vi "Ecal.vi"(0 "VISA IN":refnum<visa-resource-name>="GPIB1::16::INSTR", 5 "error in":errorcluster) -> (14 "VISA Out":refnum<visa-resource-name>="GPIB1::16::INSTR", 19 "error out":errorcluster)   [LabVIEW 2018, in "PNA-X.lvlib"]
doc: "' Performing a 2-port cal (Ports 1 and 2)\nDim app\nDim scpi\n\n' Create / Get the PNA application.\nSet app = CreateObject(\"AgilentPNA835x.Application\")\nSet scpi = app.ScpiStringParser\n\n' Specify the DUT connectors\n' (for each connector of your DUT, one of the ECal module's ports must have\n' that same connector, or else you cannot achieve the cal using that module).\nscpi.Execute \"sens:corr:coll:guid:conn:port1 \"\"APC 3.5 female\"\" \"\nscpi.Execute \"sens:corr:coll:guid:conn:port2 \"\"APC 3.5 male\"\" \"\n\n' Note: If your PNA has more than 2 ports, you would need to uncomment\n' one or both of these next two lines, to explicitly specify this is\n' just a 2-port cal.\n'scpi.Execute \"sens:corr:coll:guid:conn:port3 \"\"Not used\"\" \"\n'scpi.Execute \"sens:corr:coll:guid:conn:port4 \"\"Not used\"\" \"\nMsgBox \"Connectors defined for Ports 1 and 2\" \n\n' Select the ECal module for each port being calibrated.\n' Replace N4691-60004 with the part number printed on your module\n' followed by User x if using a User characterization, then the word 'ECal'\n' Your ECal module must already be connected via USB to the PNA.\nscpi.Execute \"sens:corr:coll:guid:ckit:port1 \"\"N4691-60004 ECal\"\" \"\nscpi.Execute \"sens:corr:coll:guid:ckit:port2 \"\"N4691-60004 User 1 ECal\"\" \"\nMsgBox \"Cal kits defined for Ports 1 and 2\"\n\n' Initiate the calibration and query the number of steps\nscpi.Execute \"sens:corr:coll:guid:init\"\nnumSteps = scpi.Execute(\"sens:corr:coll:guid:steps?\")\nMsgBox \"Number of steps is \" + CStr(numSteps)\n\n' Measure the standards\nFor i = 1 To numSteps\nstep = \"Step \" + CStr(i) + \" of \" + CStr(numSteps)\nstrPrompt = scpi.Execute(\"sens:corr:coll:guid:desc? \" + CStr(i))\nMsgBox strPrompt, vbOKOnly, step\nscpi.Execute \"sens:corr:coll:guid:acq STAN\" + CStr(i)\nNext\n\n' Conclude the calibration\nscpi.Execute \"sens:corr:coll:guid:save\"\nMsgBox \"Cal is done!\""
uses:
  PNA-X.lvlib
panel:
  in  "Orientation\nOff/On":bool=TRUE
  out "STEP":i32=1
  out "Steps":i32=1
  in  "EcalModID":string[](array[string])=["N4691-60004 ECal", "N4691-60004 ECal"]
  in  "PortConType":string[](array[string])=["APC 3.5 female", "APC 3.5 male", "Not used", "Not used"]
  in  "Channel":i32=1
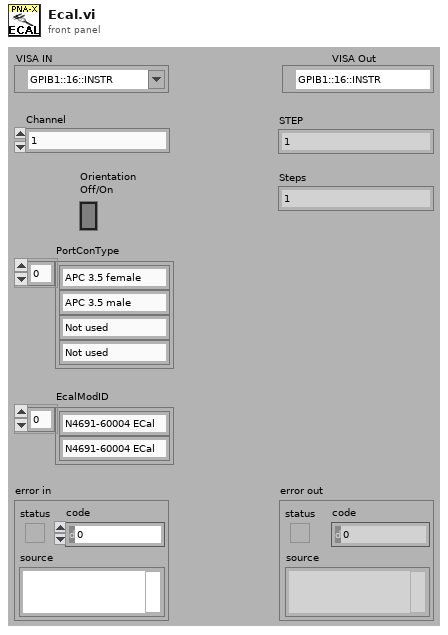
[diagram p1: front panel]
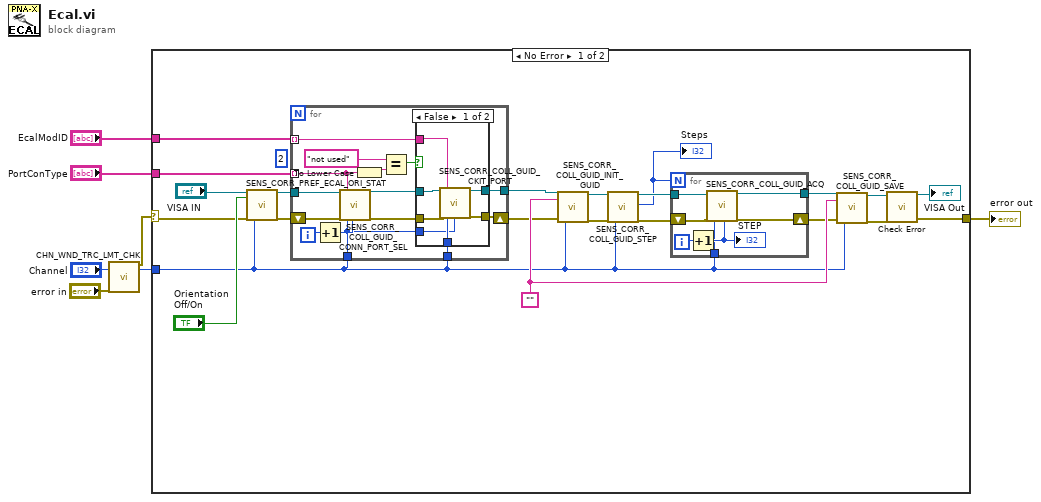
[diagram p0: block diagram]
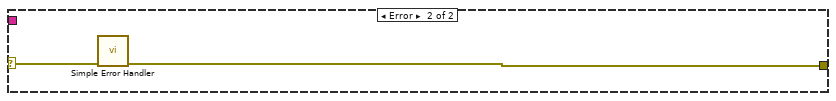
[diagram p3: hidden frame]
diagram:
  n1 = call "CHN_WND_TRC_LMT_CHK.vi"("Channel"="Channel", "error in"="error in") -> ("error out"=w1:errorcluster, "Channel"=w4:i32)  [unwired: 13 in, 3 out]
  n2 = case shown="No Error" w1 {
    selector: w1 -> [w16 w61]
    tunnel: [w22 w62] -> w2
    tunnel: "PortConType" -> [w9 _]
    tunnel: "EcalModID" -> [w10 _]
    tunnel: w4 -> [w8 _]
    frame No Error {
      (unwired) 2
      w20 = ""
      n3 = call "SENS_CORR_PREF_ECAL_ORI_STAT.vi"("VISA IN"="VISA IN", "On/Off"="Orientation\nOff/On", "error in"=w16, "Channel"=w8) -> ("VISA Out"=w13:refnum<visa-resource-name>, "error out"=w14:errorcluster)  [unwired: 14 in]
      n4 = for {
        tunnel: w13 -> [w43]
        tunnel: w9 -> [w40] mode=indexing
        shift-right: [w35] -> w11
        shift-left: w14 -> [w44]
        tunnel: [w33] -> w12
        tunnel: w10 -> [w32] mode=indexing
        tunnel: w8 -> [w30]
        tunnel: w8 -> [w31]
        i -> [w42]
        n5 = Increment(x=w42) -> (x+1=w41:i32)
        n6 = call "SENS_CORR_COLL_GUID_CONN_PORT_SEL.vi"("VISA IN"=w43, "error in"=w44, "Port Type"=w40, "Channel"=w30, "Port"=w41) -> ("VISA Out"=w34:refnum<visa-resource-name>, "error out"=w36:errorcluster)  [unwired: 13 in]
        n7 = To Lower Case(string=w40) -> (all lower case string=w39:string)
        n8 = Equal?(x="not used", y=w39) -> (x = y?=w37:bool)
        n9 = case shown="False" w37 {
          tunnel: w36 -> [w51 w52]
          tunnel: [w50 w52] -> w35
          tunnel: w34 -> [w49 w53]
          tunnel: [w48 w53] -> w33
          tunnel: w32 -> [w47 _]
          tunnel: w31 -> [w46 _]
          tunnel: w30 -> [w45 _]
          frame False {
            n10 = call "SENS_CORR_COLL_GUID_CKIT_PORT.vi"("VISA IN"=w49, "error in"=w51, "Ecal ID"=w47, "Channel"=w46, "Port"=w45) -> ("VISA Out"=w48:refnum<visa-resource-name>, "error out"=w50:errorcluster)  [unwired: 13 in]
          }
          frame True {
          }
        }
      }
      n11 = call "SENS_CORR_COLL_GUID_INIT_GUID.vi"("VISA IN"=w12, "Calset"=w20, "error in"=w11, "Channel"=w8) -> ("VISA Out"=w28:refnum<visa-resource-name>, "error out"=w21:errorcluster)  [unwired: 14 in]
      n12 = call "SENS_CORR_COLL_GUID_STEP.vi"("VISA IN"=w28, "error in"=w21, "Channel"=w8) -> ("VISA Out"=w26:refnum<visa-resource-name>, "Data"=w25:i32, "error out"=w27:errorcluster)  [unwired: 14 in]
      "Steps" <- w25
      n13 = for {
        N: w25 -> [_]
        tunnel: w26 -> [w60]
        tunnel: w8 -> [w56]
        shift-right: [w55] -> w19
        shift-left: w27 -> [w59]
        tunnel: [w54] -> w18
        i -> [w58]
        n14 = Increment(x=w58) -> (x+1=w57:i32)
        "STEP" <- w57
        n15 = call "SENS_CORR_COLL_GUID_ACQ.vi"("VISA IN"=w60, "error in"=w59, "Channel"=w56, "Standerd"=w57) -> ("VISA Out"=w54:refnum<visa-resource-name>, "error out"=w55:errorcluster)  [unwired: 14 in]
      }
      n16 = call "SENS_CORR_COLL_GUID_SAVE.vi"("VISA IN"=w18, "Calset"=w20, "error in"=w19, "Channel"=w8) -> ("VISA Out"=w23:refnum<visa-resource-name>, "error out"=w24:errorcluster)  [unwired: 14 in]
      n17 = call "Check Error.vi"("VISA Resource Name"=w23, "error in (no error)"=w24) -> ("dup VISA session"=→"VISA Out":refnum<visa-resource-name>, "error out"=w22:errorcluster)  [unwired: 16 in]
    }
    frame Error {
      n18 = call <vilib>:"Simple Error Handler.vi"("error in (no error)"=w61) -> ("error out"=w62:errorcluster)  [unwired: 4 in, 4 out]
    }
  }
  "error out" <- w2
